vi "Angle.vi"(10 "B":refnum<class "Vector 2D.lvclass">, 11 "A":refnum<class "Vector 2D.lvclass">) -> (3 "Angle [deg]":dbl)   [LabVIEW 2021, in "Vector 2D.lvclass"]
uses:
  Vector 2D.lvclass
  Vector 2D.lvclass/Vector 2D.ctl
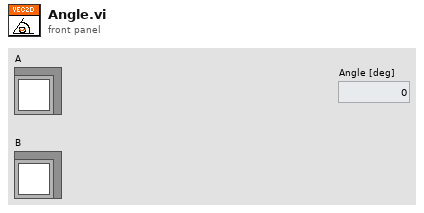
[diagram p1: front panel]
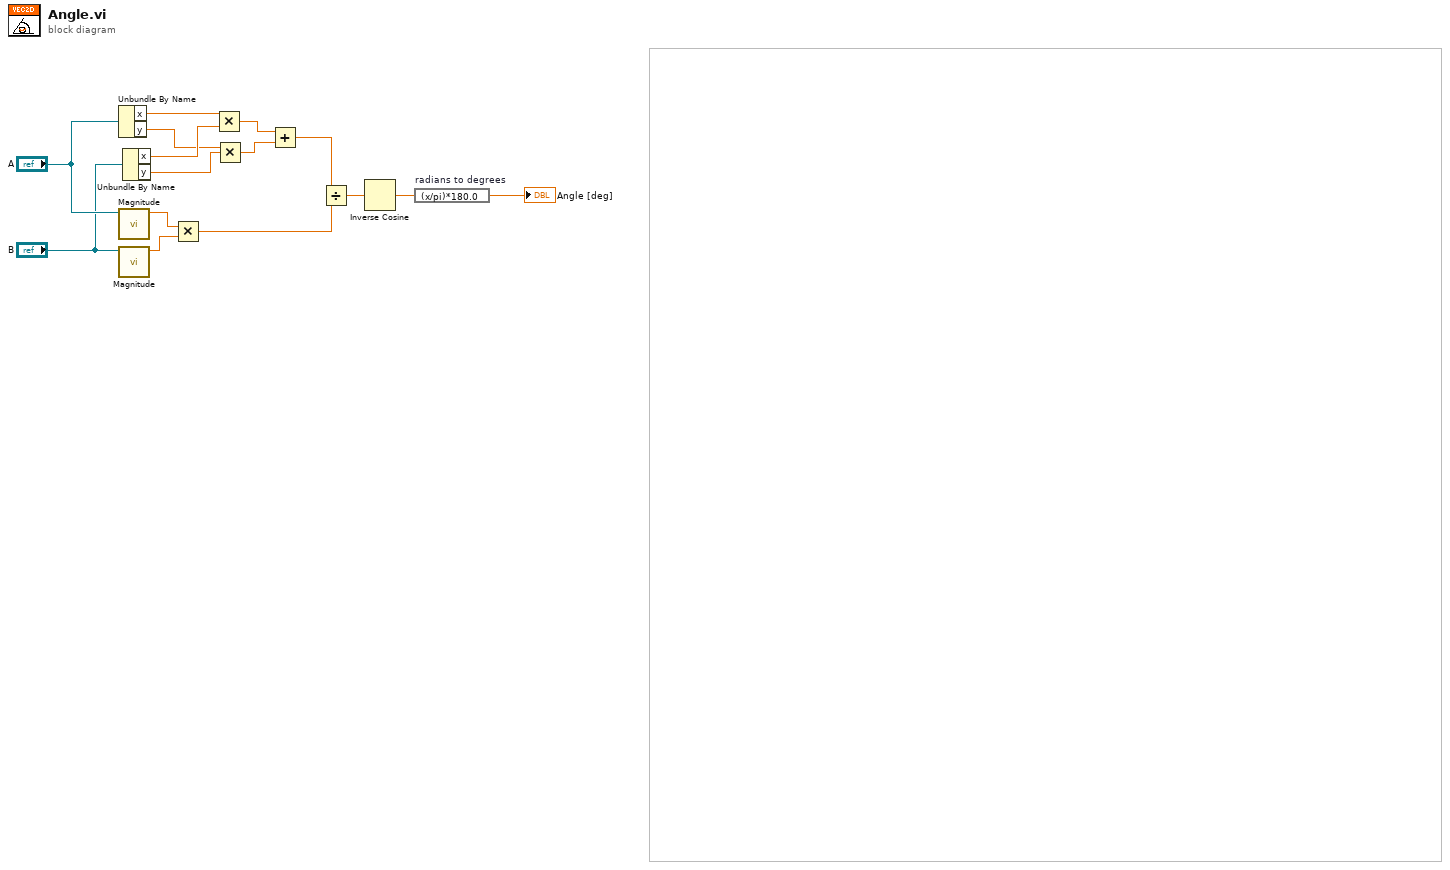
[diagram p0: block diagram]
diagram:
  n1 = Unbundle By Name("A") -> ("x"=w13:sgl, "y"=w4:sgl)
  n2 = call "Magnitude.vi"("A"="A") -> ("Magnitude"=w10:sgl)  [unwired: 10 in]
  n3 = call "Magnitude.vi"("A"="B") -> ("Magnitude"=w9:sgl)  [unwired: 10 in]
  n4 = Unbundle By Name("B") -> ("x"=w5:sgl, "y"=w3:sgl)
  n5 = Multiply(x=w10, y=w9) -> (x*y=w7:sgl)
  n6 = Multiply(x=w13, y=w5) -> (x*y=w12:sgl)
  n7 = Multiply(x=w4, y=w3) -> (x*y=w11:sgl)
  n8 = Add(x=w12, y=w11) -> (x+y=w8:sgl)
  n9 = Divide(x=w8, y=w7) -> (x/y=w6:sgl)
  n10 = Inverse Cosine(1:w6) -> (0:w2:sgl)
  n11 = expression code="(x/pi)*180.0" "radians to degrees"(w2) -> (→"Angle [deg]":sgl)
